vi "2023 Teleop Arm Control.vi"() -> (1 "Commanded\nSet Output":dbl, 2 "Current":dbl, 3 "Sensor Velocity":dbl, 4 "Sensor Position":dbl)   [LabVIEW 2020]
uses:
  <vilib>/Rock Robotics/WPI/ThirdParty/Phoenix-LabVIEW/Motor Controller/Controls/CTRE_Phoenix_MotorControl_ControlMode.ctl
  <vilib>/Rock Robotics/WPI/Utilities/WPI_GetSetVariantRefNum.vi
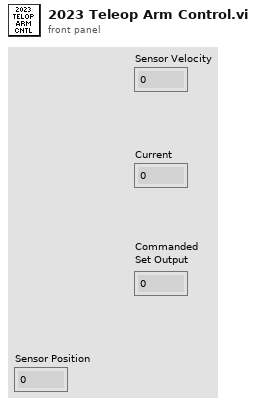
[diagram p1: front panel]
types:
  T1 = typedef "CTRE_Phoenix_MotorControl_ControlMode.ctl" = u16
  T2 = typedef "WPI_JoystickDevRef.ctl" = cluster{"Device":T3}
  T3 = typedef "WPI_JoystickDeviceEnum.ctl" = enum16{"USB 0", "USB 1", "USB 2", "USB 3", "USB 4", "USB 5"}
  T4 = typedef "WPI_MotorControlDeviceRef.ctl" = cluster{"DeviceStatus":errorcluster, "Type":T5, "PWM":cluster{"PWM Channel":T6, "DeadBand":T7}, "CAN":cluster{"Device Number":u8, "SetOutput VI Ref":variant, "GetOutput VI Ref":variant, "Enable VI Ref":variant, "Disable VI Ref":variant, "Data":variant}, "Invert":bool, "DIO PWM":cluster{"PWM \"Enable\" Channel":T6, "DIOChannel":T8, "PWM Rate":dbl}}
  T5 = typedef "WPI_MotorControlType.ctl" = enum16{"PWM", "CAN", "DIO PWM"}
  T6 = typedef "FPGA_DIOPWMChannel.ctl" = enum8{"PWM 0", "PWM 1", "PWM 2", "PWM 3", "PWM 4", "PWM 5", "PWM 6", "PWM 7", "PWM 8", "PWM 9", "PWM MXP 0", "PWM MXP 1", "PWM MXP 2", "PWM MXP 3", "PWM MXP 4", "PWM MXP 5", "PWM MXP 6", "PWM MXP 7", "PWM MXP 8", "PWM MXP 9", "Invalid"}
  T7 = typedef "WPI_PWMDeadband.ctl" = cluster{"Name":string, "maxPositivePwm":i32, "minPositivePwm":i32, "centerPwm":i32, "maxNegativePwm":i32, "minNegativePwm":i32, "angularRange":u16}
  T8 = typedef "FPGA_DIOChannel.ctl" = enum8{"DIO 0", "DIO 1", "DIO 2", "DIO 3", "DIO 4", "DIO 5", "DIO 6", "DIO 7", "DIO 8", "DIO 9", "DIO MXP 0", "DIO MXP 1", "DIO MXP 2", "DIO MXP 3", "DIO MXP 4", "DIO MXP 5", "DIO MXP 6", "DIO MXP 7", "DIO MXP 8", "DIO MXP 9", "DIO MXP 10", "DIO MXP 11", "DIO MXP 12", "DIO MXP 13", "DIO MXP 14", "DIO MXP 15", "SPI Port CS1", "SPI Port CS2", "SPI Port CS3", "SPI Port MISO", "SPI Port MOSI", "Invalid"}
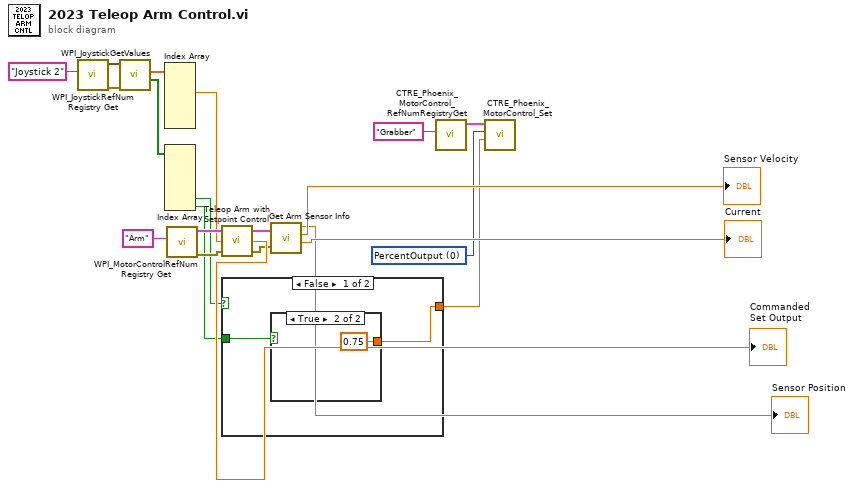
[diagram p0: block diagram]
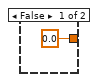
[diagram p2: hidden frame]
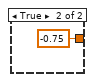
[diagram p3: hidden frame]
diagram:
  w12 = T1 0 items=["PercentOutput"=0, "Position"=1, "Velocity"=2, "Current"=3, "Follower"=5, "MotionProfile"=6, "MotionMagic"=7, "MotionProfileArc"=10, "Disabled"=15] ("Control Mode")
  n1 = call <vilib>:"WPI_JoystickRefNum Registry Get.vi"("refnum name"="Joystick 2") -> ("error out"=w5:errorcluster, "JoystickDevRef"=w4:T2)  [unwired: 1 in, 8 out]
  n2 = call <vilib>:"WPI_JoystickGetValues.vi"("error in (no error)"=w5, "JoystickDevRef"=w4) -> ("Buttons"=w6:bool[], "Axes"=w9:dbl[])  [unwired: 5 in, 3 out]
  n3 = Index Array(array=w9) -> (element #2=w13:dbl)  [unwired: 6 in, 5 out]
  n4 = Index Array(array=w6) -> (element #5=w7:bool, element #6=w8:bool)  [unwired: 6 in, 4 out]
  n5 = call <vilib>:"WPI_MotorControlRefNum Registry Get.vi"("refnum name"="Arm") -> ("error out"=w15:errorcluster, "MotorControlDevRef"=w14:T4)  [unwired: 9 in]
  n6 = call "Teleop Arm with Setpoint Control.vi"("error in (no error)"=w15, "Joystick Command"=w13, "MotorControlDevRef"=w14) -> ("error out"=w17:errorcluster, "Commanded\nSet Output"=→"Commanded\nSet Output":dbl, "MotorControlOutput"=w16:T4)
  n7 = case shown="False" w7 {
    tunnel: [w22 -0.75] -> w10
    tunnel: w8 -> [w23 _]
    frame False {
      n8 = case shown="True" w23 {
        tunnel: [0.0 0.75] -> w22
        frame False {
        }
        frame True {
        }
      }
    }
    frame True {
    }
  }
  n9 = call "Get Arm Sensor Info.vi"("MotorControlDevRef"=w16, "error in (no error)"=w17) -> ("Sensor Position"=→"Sensor Position":dbl, "Sensor Velocity"=→"Sensor Velocity":dbl, "Current"=→"Current":dbl)  [unwired: 1 out]
  n10 = call <vilib>:"CTRE_Phoenix_MotorControl_RefNumRegistryGet.vi"("refnum name"="Grabber") -> ("PhoenixMotorControlDevRef"=w1:T4)  [unwired: 9 in, 1 out]
  n11 = call <vilib>:"CTRE_Phoenix_MotorControl_Set.vi"("Output"=w10, "Control Mode"=w12, "PhoenixMotorControlDevRef"=w1) -> ()  [unwired: 7 in, 2 out]
